vi "Win_PCAN_Config.vi"(8 "error in":errorcluster caption="错误输入") -> (0 "error out":errorcluster caption="错误输出", 1 "FilterMessages":cluster{"Mode: ":T1, "From:":u32, "To:":u32}={"Mode: "=0, "From:"=0, "To:"=2047} {"To:" format="%.0x"; "From:" format="%.0x"; "Mode:" items=["PCAN_MODE_STANDARD"=0, "PCAN_MODE_EXTENDED"=2]}, 2 "Initialize":cluster{"Bit rate:":T3, "HwType: ":T2}={"Bit rate:"=28, "HwType: "=1} {"HwType:" items=["PCAN_TYPE_ISA"=1, "PCAN_TYPE_ISA_SJA"=9, "PCAN_TYPE_ISA_PHYTEC"=4, "PCAN_TYPE_DNG"=2, "PCAN_TYPE_DNG_EPP"=3, "PCAN_TYPE_DNG_SJA"=5, "PCAN_TYPE_DNG_SJA_EPP"=6]; "Bit rate:" items=["PCAN_BAUD_1M"=20, "PCAN_BAUD_800K"=22, "PCAN_BAUD_500K"=28, "PCAN_BAUD_250K"=284, "PCAN_BAUD_125K"=796]}, 3 "Channel out":T4=81 items=["PCAN_USBBUS1"=81, "PCAN_USBBUS2"=82, "PCAN_USBBUS3"=83, "PCAN_USBBUS4"=84], 4 "Yes out":bool=TRUE)   [LabVIEW 2020]
uses:
  Control/Channel.ctl
  Control/Bit rate.ctl
  Control/HwType.ctl
  Control/Mode.ctl
  <vilib>/Utility/xml.llb/Write to XML File(array).vi
panel:
  in  "Mode:":T1 items=["PCAN_MODE_STANDARD"=0, "PCAN_MODE_EXTENDED"=2]
  in  "HwType:":T2=1 items=["PCAN_TYPE_ISA"=1, "PCAN_TYPE_ISA_SJA"=9, "PCAN_TYPE_ISA_PHYTEC"=4, "PCAN_TYPE_DNG"=2, "PCAN_TYPE_DNG_EPP"=3, "PCAN_TYPE_DNG_SJA"=5, "PCAN_TYPE_DNG_SJA_EPP"=6]
  in  "Bit rate:":T3=28 items=["PCAN_BAUD_1M"=20, "PCAN_BAUD_800K"=22, "PCAN_BAUD_500K"=28, "PCAN_BAUD_250K"=284, "PCAN_BAUD_125K"=796]
  in  "To:":u32=2047 format="%.0x"
  in  "From:":u32 format="%.0x"
  in  "No":bool
  in  "Yes":bool
  in  "Channel:":T4=81 items=["PCAN_USBBUS1"=81, "PCAN_USBBUS2"=82, "PCAN_USBBUS3"=83, "PCAN_USBBUS4"=84]
  # "Filter settings"
  # "(Hex)"
  # "(Hex)"
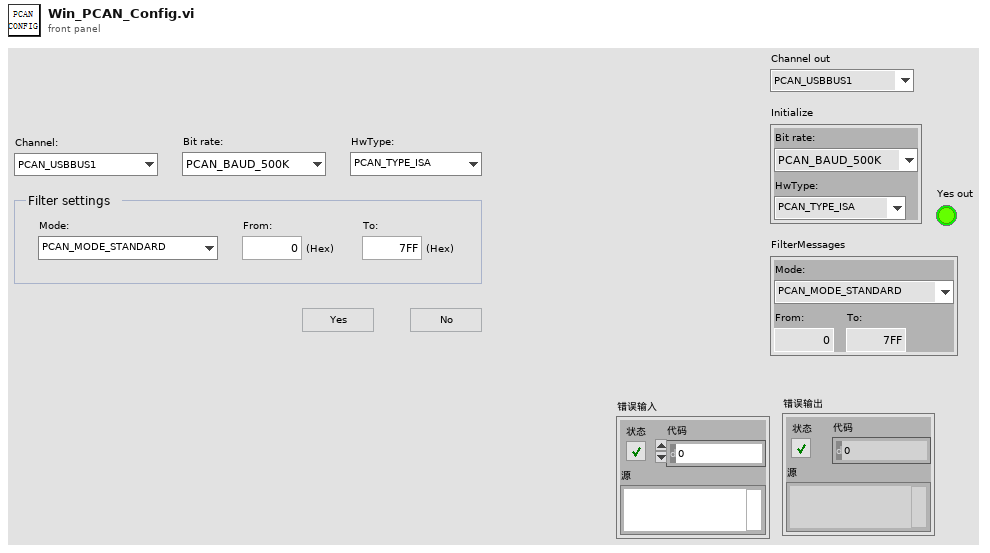
[diagram p1: front panel]
types:
  T1 = typedef "Mode.ctl" = u8
  T2 = typedef "HwType.ctl" = u8
  T3 = typedef "Bit rate.ctl" = u16
  T4 = typedef "Channel.ctl" = u16
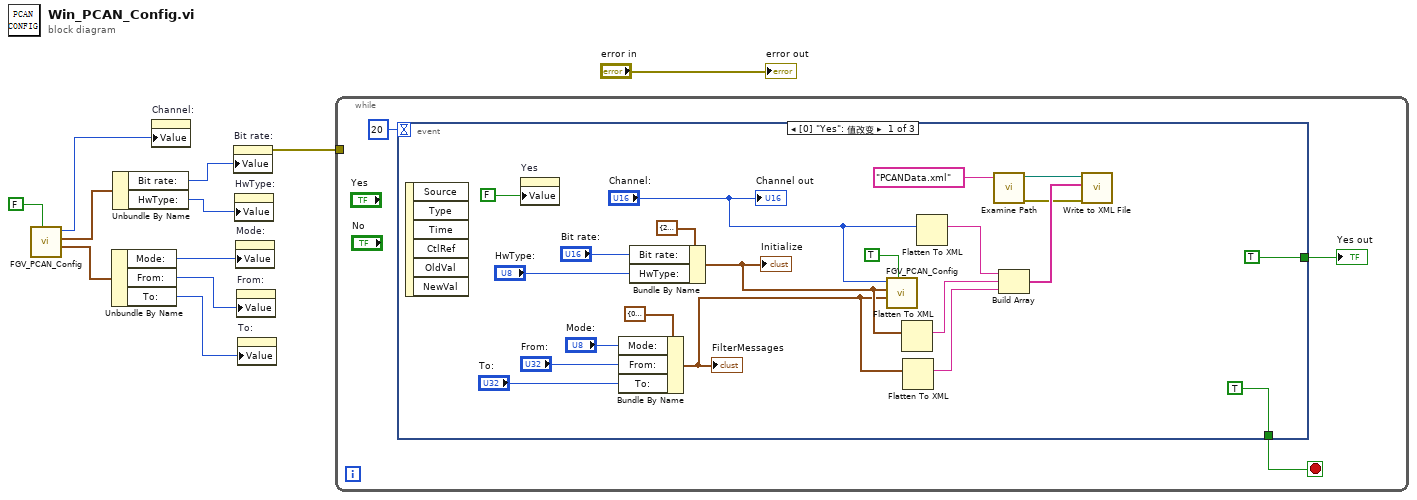
[diagram p0: block diagram]
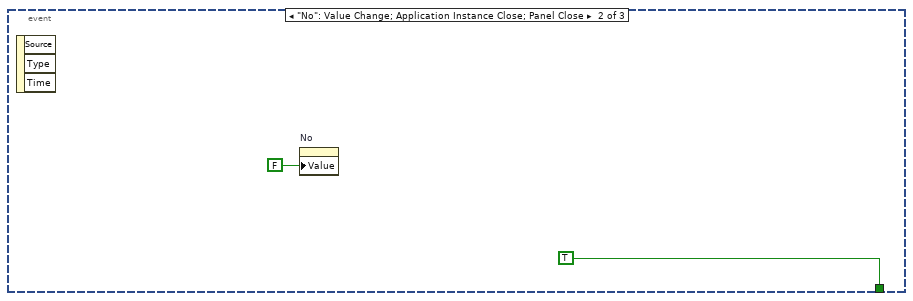
[diagram p2: hidden frame]
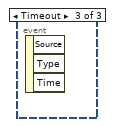
[diagram p3: hidden frame]
diagram:
  n1 = call "FGV_PCAN_Config.vi"("Write?"=FALSE) -> ("FilterMessages out"=w6:cluster{"Mode: ":T1, "From:":u32, "To:":u32}, "Initialize out"=w7:cluster{"Bit rate:":T3, "HwType: ":T2}, "Channel out"=w8:T4)  [unwired: 7 in, 1 out]
  n2 = Unbundle By Name(w6) -> ("Mode:"=w3:T1, "From:"=w2:u32, "To:"=w1:u32)
  n3 = Unbundle By Name(w7) -> ("Bit rate:"=w5:T3, "HwType:"=w4:T2)
  n4 = property on="Channel:" class="Ring (严格)"("Value"=w8) -> ()  [unwired: 2 in, 2 out]
  n5 = property on="Bit rate:" class="Ring (严格)"("Value"=w5) -> (error out=w10:errorcluster)  [unwired: 2 in, 1 out]
  n6 = property on="HwType:" class="Ring (严格)"("Value"=w4) -> ()  [unwired: 2 in, 2 out]
  n7 = property on="Mode:" class="Ring (严格)"("Value"=w3) -> ()  [unwired: 2 in, 2 out]
  n8 = property on="From:" class="DigNum (严格)"("Value"=w2) -> ()  [unwired: 2 in, 2 out]
  n9 = property on="To:" class="DigNum (严格)"("Value"=w1) -> ()  [unwired: 2 in, 2 out]
  n10 = while {
    tunnel: w10 -> [_]
    stop <- w13 stop-if-true
    n11 = event shown="[0] \"Yes\": 值改变" {
      selector: _ -> [_ _ _]
      dyn-events: _ -> [_ _ _]
      timeout: 20 -> [_ _ _]
      tunnel: [TRUE TRUE _] -> w13
      tunnel: [TRUE _ _] -> w12
      event "Yes": Value Change {
        n12 = event-data() -> ()  [unwired: 1 in, 6 out]
        n13 = property on="Yes" class="Bool (严格)"("Value"=FALSE ("Yes")) -> ()  [unwired: 2 in, 2 out]
        n14 = Bundle By Name(cluster=cluster{"Mode: ":T1, "From:":u32, "To:":u32} {"Mode: "=0, "From:"=0, "To:"=0} ("FilterMessages"), "Mode:"="Mode:", "From:"="From:", "To:"="To:") -> (w21:cluster{"Mode: ":T1, "From:":u32, "To:":u32})
        "FilterMessages" <- w21
        n15 = Bundle By Name(cluster=cluster{"Bit rate:":T3, "HwType: ":T2} {"Bit rate:"=28, "HwType: "=1} ("Initialize"), "Bit rate:"="Bit rate:", "HwType:"="HwType:") -> (w22:cluster{"Bit rate:":T3, "HwType: ":T2})
        "Initialize" <- w22
        n16 = call "FGV_PCAN_Config.vi"("Write?"=TRUE, "FilterMessages"=w21, "Initialize"=w22, "Channel"="Channel:") -> ()  [unwired: 4 in, 4 out]
        n17 = Flatten To XML(6:w22) -> (2:w19:string)
        n18 = Flatten To XML(6:w21) -> (2:w18:string)
        n19 = Flatten To XML(6:"Channel:") -> (2:w20:string)
        n20 = call "Examine Path.vi"("Filename"="PCANData.xml") -> ("error out"=w15:errorcluster, "Path"=w17:path)  [unwired: 9 in]
        n21 = Build Array(w20, w19, w18) -> (w16:string[])
        n22 = call-poly <vilib>:"Write to XML File.vi"("error in (no error)"=w15, "XML Input"=w16, "XML File Path"=w17) -> ()  [unwired: 6 in, 3 out]
        "Channel out" <- "Channel:"
      }
      event "No": Value Change; Application Instance Close; Panel Close {
        n23 = event-data() -> ()  [unwired: 1 in, 3 out]
        n24 = property on="No" class="Bool (严格)"("Value"=FALSE ("No")) -> ()  [unwired: 2 in, 2 out]
      }
      event Timeout {
        n25 = event-data() -> ()  [unwired: 1 in, 3 out]
      }
    }
    "Yes out" <- w12
  }
  "error out" <- "error in"
